vi "OAT Convert Phase (N Channels).vi"(6 "input unit in degree?":bool, 7 "reset (TRUE)":bool=TRUE, 10 "desired phase setting":T1, 11 "phase in":dbl[][][](array[numeric]) format="%.2f") -> (3 "phase out":dbl[][][](array[numeric]) format="%.2f")   [LabVIEW 2017]
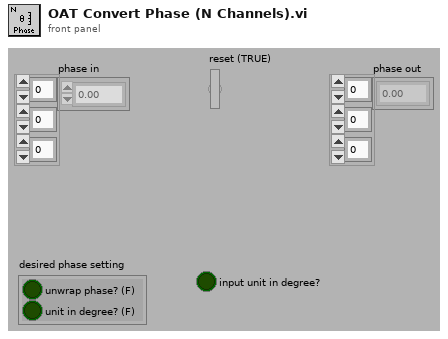
[diagram p1: front panel]
types:
  T1 = cluster{"unwrap phase? (F)":bool, "unit in degree? (F)":bool}
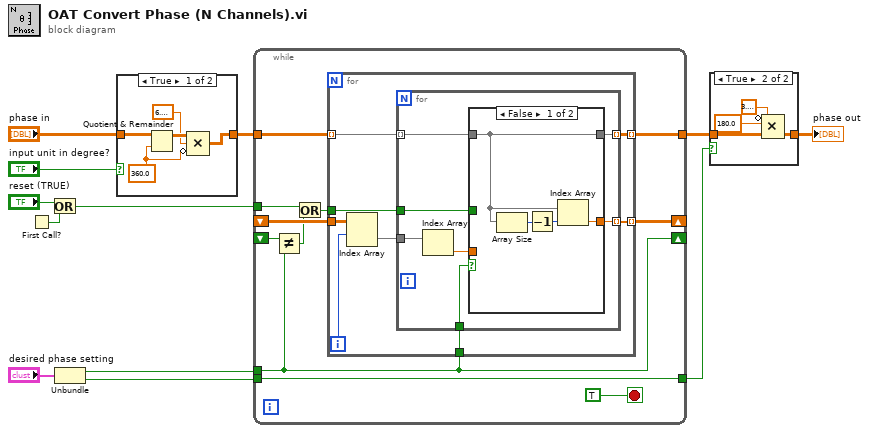
[diagram p0: block diagram]
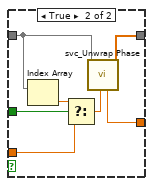
[diagram p2: hidden frame]
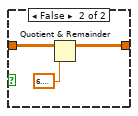
[diagram p4: hidden frame]
diagram:
  n1 = First Call?() -> (First Call?: T/F=w11:bool)
  n2 = Or(x="reset (TRUE)", y=w11) -> (x .or. y?=w10:bool)
  n3 = Unbundle("desired phase setting") -> ("unwrap phase? (F)"=w9:bool, "unit in degree? (F)"=w8:bool)
  n4 = case shown="True" "input unit in degree?" {
    tunnel: "phase in" -> [w17 w19]
    tunnel: [w13 w18] -> w6
    frame True {
      w14 = 360.0
      n5 = Quotient & Remainder(x=w17, y=w14) -> (x-y*floor(x/y)=w16:dbl[][][])  [unwired: 1 out]
      n6 = Compound Arithmetic op=MULTIPLY(w16, 6.283185307179586, invert w14) -> (w13:dbl[][][])
    }
    frame False {
      n7 = Quotient & Remainder(x=w19, y=6.283185307179586) -> (x-y*floor(x/y)=w18:dbl[][][])  [unwired: 1 out]
    }
  }
  n8 = while {
    tunnel: [w22] -> w4
    tunnel: w9 -> [w27]
    tunnel: w8 -> [w21]
    tunnel: w6 -> [w31]
    shift-right: [w28] -> _
    shift-left: _ -> [w29]
    tunnel: w10 -> [w25]
    shift-right: [w27] -> _
    shift-left: _ -> [w23]
    tunnel: [w21] -> w3
    stop <- TRUE stop-if-true
    n9 = Not Equal?(x=w23, y=w27) -> (x != y?=w26:bool)
    n10 = Or(x=w25, y=w26) -> (x .or. y?=w24:bool)
    n11 = for {
      tunnel: [w36] -> w22 mode=indexing
      tunnel: w27 -> [w33]
      tunnel: w31 -> [w38] mode=indexing
      tunnel: w29 -> [w39]
      tunnel: w24 -> [w37]
      tunnel: [w35] -> w28 mode=indexing
      i -> [w32]
      n12 = Index Array(array=w39, index (row)=w32) -> (element=w34:dbl[])  [unwired: 1 in]
      n13 = for {
        tunnel: [w44] -> w36 mode=indexing
        tunnel: w33 -> [w40]
        tunnel: w38 -> [w46] mode=indexing
        tunnel: w34 -> [w42]
        tunnel: w37 -> [w43]
        tunnel: [w45] -> w35 mode=indexing
        n14 = Index Array(array=w42) -> (element=w41:dbl)  [unwired: 1 in]
        n15 = case shown="False" w40 {
          tunnel: [w50 w53] -> w44
          tunnel: w46 -> [w50 w54]
          tunnel: [w47 w51] -> w45
          tunnel: w41 -> [_ w56]
          tunnel: w43 -> [_ w55]
          frame False {
            n16 = Array Size(array=w50) -> (size(s)=w49:i32)
            n17 = Decrement(x=w49) -> (x-1=w48:i32)
            n18 = Index Array(array=w50, index=w48) -> (element=w47:dbl)
          }
          frame True {
            n19 = Index Array(array=w54) -> (element=w57:dbl)  [unwired: 1 in]
            n20 = Select(t=w57, s=w55, f=w56) -> (s? t:f=w52:dbl)
            n21 = call <vilib>:"svc_Unwrap Phase.vi"("start phase"=w52, "phase in"=w54) -> ("phase out"=w53:dbl[], "end phase"=w51:dbl)  [unwired: 8 in]
          }
        }
      }
    }
  }
  n22 = case shown="True" w3 {
    tunnel: w4 -> [w58 w60]
    tunnel: [w58 w59] -> w2
    frame False {
    }
    frame True {
      n23 = Compound Arithmetic op=MULTIPLY(invert 3.141592653589793, 180.0, w60) -> (w59:dbl[][][])
    }
  }
  "phase out" <- w2
